vi "Message analysis.vi"(10 "DBMessage":T1 {"BRS" items=["No BRS", "BRS"]; "ID" format="%.0x"; "Type" items=["cftStdCAN", "cftExtCAN", "cftJ1939", "cftStdCANFD", "cftExtCANFD"]}, 11 "Value in":string[][](array[string])) -> (3 "Value out":string[][](array[string]))   [LabVIEW 2014]
uses:
  Typedef/DBMessage.ctl
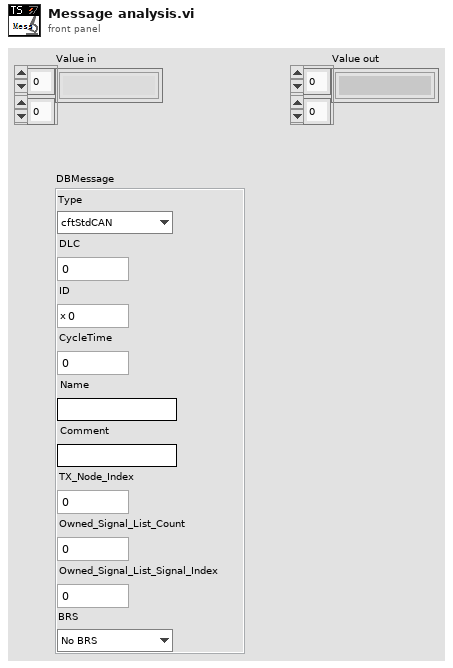
[diagram p1: front panel]
types:
  T1 = typedef "DBMessage.ctl" = cluster{"Type":u16, "DLC":i32, "ID":i32, "CycleTime":dbl, "Name":string, "Comment":string, "TX_Node_Index":i32, "Owned_Signal_List_Count ":i32, "Owned_Signal_List_Signal_Index":i32, "BRS":i32}
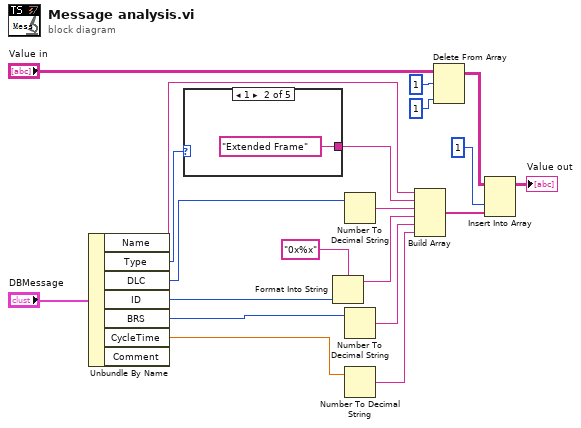
[diagram p0: block diagram]
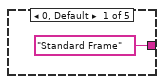
[diagram p2: hidden frame]
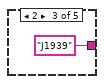
[diagram p3: hidden frame]
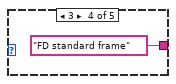
[diagram p4: hidden frame]
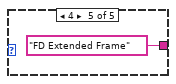
[diagram p5: hidden frame]
diagram:
  n1 = Unbundle By Name("DBMessage") -> ("Name"=w8:string, "Type"=w5:u16, "DLC"=w4:i32, "ID"=w6:i32, "BRS"=w3:i32, "CycleTime"=w2:dbl)  [unwired: 1 out]
  n2 = case shown="1" w5 {
    tunnel: ["Standard Frame" "Extended Frame" "J1939" "FD standard frame" "FD Extended Frame"] -> w9
    frame 0, Default {
    }
    frame 1 {
    }
    frame 2 {
    }
    frame 3 {
    }
    frame 4 {
    }
  }
  n3 = Format Into String(format string="0x%x", w6) -> (resulting string=w11:string)  [unwired: 2 in, 1 out]
  n4 = Number To Decimal String(number=w4) -> (decimal integer string=w10:string)  [unwired: 1 in]
  n5 = Number To Decimal String(number=w3) -> (decimal integer string=w12:string)  [unwired: 1 in]
  n6 = Number To Decimal String(number=w2) -> (decimal integer string=w13:string)  [unwired: 1 in]
  n7 = Build Array(w8, w9, w10, w11, w12, w13) -> (w19:string[])
  n8 = Delete From Array(array="Value in", length=1 ("disabled index (col)"), index (col)=1 ("disabled index (col)")) -> (array with subset deleted=w17:string[][])  [unwired: 1 in, 1 out]
  n9 = Insert Into Array(array=w17, index (col)=1 ("disabled index (col)"), new element=w19) -> (→"Value out":string[][])  [unwired: 1 in]
